vi "loadSRM.vi"() -> ()   [LabVIEW 2012]
panel:
  out "error out":cluster{"status":bool, "code":i32}
  out "String":string
  in  "Array":string[](array[string])=["192.168.1.13\\equ-summary\\hexa\\FLST08", "192.168.1.13\\equ-summary\\hexa\\FLST09", "192.168.1.13\\equ-summary\\hexa\\FLST10", "192.168.1.13\\equ-summary\\hexa\\FLST11", "192.168.1.13\\equ-summary\\hexa\\FLST12", "192.168.1.13\\equ-summary\\hexa\\FLST13", "192.168.1.13\\equ-summary\\hexa\\FLST14", "192.168.1.13\\equ-summary\\hexa\\FLST15", "192.168.1.13\\equ-summary\\hexa\\FLST21", "192.168.1.13\\equ-summary\\hexa\\FLST22", "192.168.1.13\\equ-summary\\hexa\\FLST27", "192.168.1.13\\equ-summary\\hexa\\FLST28"]
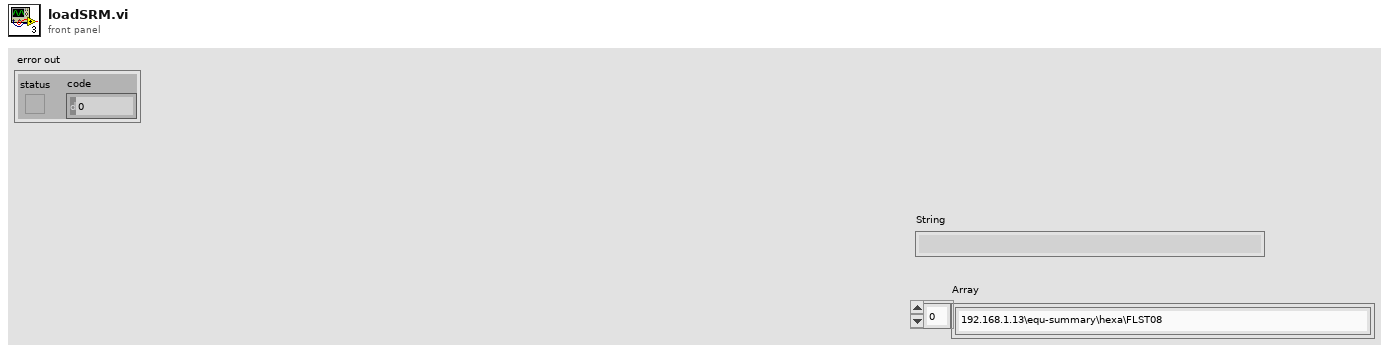
[diagram p1: front panel]
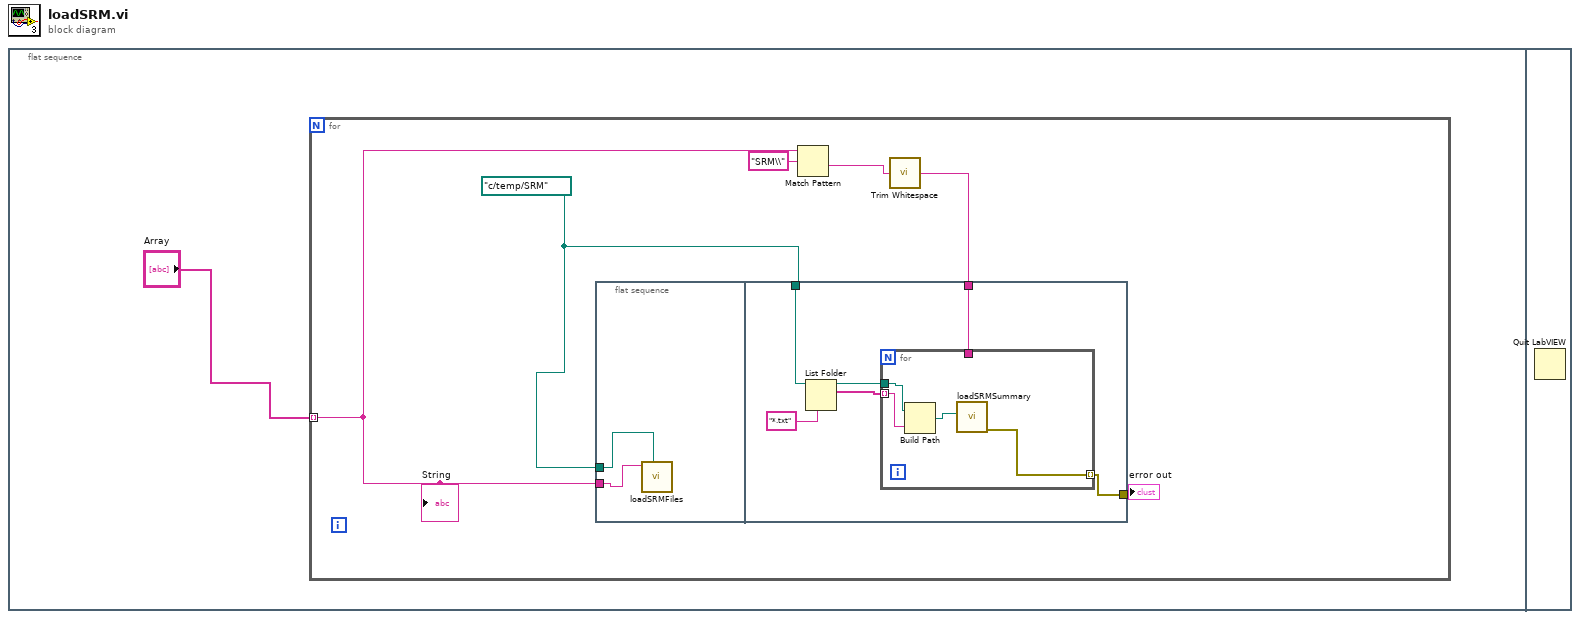
[diagram p0: block diagram]
diagram:
  n1 = flat-sequence {
    frame #0 {
      n2 = for {
        tunnel: "Array" -> [w5] mode=indexing
        w6 = path "c:/temp/SRM" ("working directory")
        n3 = flat-sequence {
          tunnel: w5 -> [w8]
          tunnel: w6 -> [w7]
          tunnel: [w14] -> _
          tunnel: w6 -> [w13]
          tunnel: w2 -> [w9]
          frame #0 {
            n4 = call "loadSRMFiles.vi"("working directory"=w7, "folder"=w8) -> ()  [unwired: 10 in]
          }
          frame #1 {
            n5 = List Folder(path=w13, pattern="*.txt") -> (path out=w10:path, filenames=w11:string[])  [unwired: 2 in, 2 out]
            n6 = for {
              tunnel: [w18] -> w14 mode=indexing
              tunnel: w11 -> [w16] mode=indexing
              tunnel: w10 -> [w15]
              tunnel: w9 -> [_]
              n7 = Build Path(base path=w15, name or relative path=w16) -> (appended path=w17:path)
              n8 = call "loadSRMSummary.vi"("file path (dialog if empty)"=w17) -> ("error out"=w18:errorcluster)  [unwired: 10 in]
            }
          }
        }
        n9 = Match Pattern(string=w5, regular expression="SRM\\") -> (after substring=w3:string)  [unwired: 1 in, 3 out]
        n10 = call <vilib>:"Trim Whitespace.vi"("string"=w3) -> ("trimmed string"=w2:string)  [unwired: 1 in]
        "String" <- w5
      }
    }
    frame #1 {
      n11 = Quit LabVIEW() -> ()  [unwired: 1 in]
    }
  }
